vi "Test Case, Read-Write Waveform File.vi"() -> ()   [LabVIEW 2010]
panel:
  in  "error in":errorcluster
  out "error out":errorcluster
  out "date and time out":timestamp=timestamp(-9593226000 s since 1904-01-01) format="%<%.1X  %x>T "
  out "date and time in":timestamp format="%<%.1X  %x>T"
  out "waveform out":waveform(dbl)={"t0"=timestamp(0 s since 1904-01-01), "dt"=nan, "Y"=[]}
  out "WF data\n x = y?":bool
  in  "waveform in":waveform(dbl)={"t0"=timestamp(2230740000 s since 1904-01-01), "dt"=1.0, "Y"=[1.0, 2.0, 3.0]}
  in  "file path":path=path "c:/temp.dat"
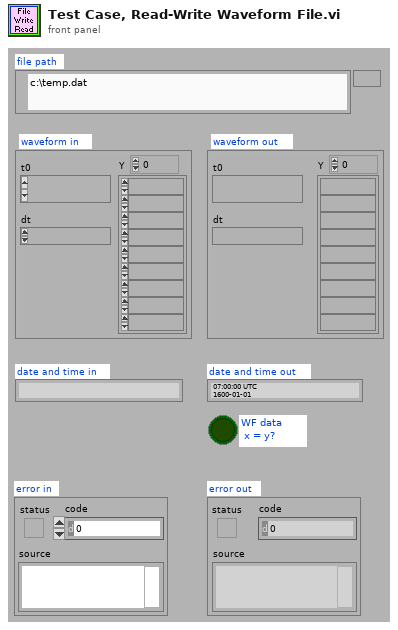
[diagram p1: front panel]
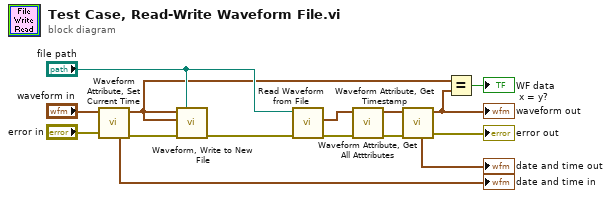
[diagram p0: block diagram]
diagram:
  n1 = call "Waveform Attribute, Set Current Time.vi"("error in"="error in", "waveform"="waveform in") -> ("error out"=w13:errorcluster, "waveform out"=w1:waveform(dbl), "Date and Time"=→"date and time in":timestamp)  [unwired: 4 in, 1 out]
  n2 = call "Waveform, Write to New File.vi"("filepath"="file path", "error in"=w13, "prc waveform"=w1, "raw waveform"=w1) -> ("error out"=w14:errorcluster)  [unwired: 2 in, 3 out]
  n3 = call <vilib>:"Read Waveform from File.vi"("error in (no error)"=w14, "file path (dialog if empty)"="file path") -> ("error out"=w10:errorcluster, "first waveform in record"=w11:waveform(dbl))  [unwired: 4 in, 2 out]
  n4 = call "Waveform Attribute, Get All Atttributes.vi"("error in"=w10, "waveform"=w11) -> ("error out"=w9:errorcluster, "waveform dup"=w6:waveform(dbl))  [unwired: 5 in, 1 out]
  n5 = call "Waveform Attribute, Get Timestamp.vi"("error in"=w9, "waveform"=w6) -> ("error out"=→"error out":errorcluster, "waveform dup"=w4:waveform(dbl), "Date and Time"=→"date and time out":timestamp)  [unwired: 4 in, 1 out]
  "waveform out" <- w4
  n6 = Equal?(x=w1, y=w4) -> (x = y?=→"WF data\n x = y?":bool)
